vi "Main Target v3.vi"() -> ()   [LabVIEW 2018]
uses:
  Messages.ctl
  Target Logging Cluster.ctl
  Logging Data Cluster.ctl
  Target Logging Control Signals.ctl
  Target Logging Sensors.ctl
  Sensor Data.ctl
  <vilib>/Platform/TimedLoop/XDataNode/timing_clust.ctl
  <vilib>/Platform/TimedLoop/XDataNode/nitl_modes.ctl
  <vilib>/Platform/TimedLoop/XDataNode/wakeup.ctl
  Target IO Initialized Cluster.ctl
  <vilib>/myRIO/Instrument Drivers/Onboard IO/AI/typedefs/AI Reference.ctl
  <vilib>/myRIO/Common/Instrument Driver Framework/Utilities/typedefs/myRIO Generic Hardware Reference.ctl
  <vilib>/myRIO/Common/Instrument Driver Framework/Utilities/typedefs/Hardware Version Enum.ctl
  <vilib>/myRIO/Common/Instrument Driver Framework/Utilities/typedefs/myRIO v1.0 Reference.ctl
  <vilib>/myRIO/Common/Instrument Driver Framework/Utilities/typedefs/Generic FPGA Reference.ctl
  <vilib>/myRIO/Common/Instrument Driver Framework/myRIO v1.0/AI/typedefs/AI Channels List.ctl
  <vilib>/myRIO/Common/Instrument Driver Framework/myRIO v1.0/AI/typedefs/AI Channels Enum.ctl
  <vilib>/myRIO/Common/Instrument Driver Framework/Utilities/typedefs/Analog Scaling Constants List.ctl
  <vilib>/myRIO/Common/Instrument Driver Framework/Utilities/typedefs/Analog Scaling Constants.ctl
  <vilib>/myRIO/Instrument Drivers/Onboard IO/AO/typedefs/AO Reference.ctl
  <vilib>/myRIO/Common/Instrument Driver Framework/myRIO v1.0/AO/typedefs/AO Channels List.ctl
  <vilib>/myRIO/Common/Instrument Driver Framework/myRIO v1.0/AO/typedefs/AO Channels Enum.ctl
  <vilib>/myRIO/Instrument Drivers/Onboard IO/Encoder/typedefs/Encoder Reference.ctl
  <vilib>/myRIO/Common/Instrument Driver Framework/myRIO v1.0/Encoder/typedefs/Encoder Channels Enum.ctl
  <vilib>/myRIO/Instrument Drivers/Onboard IO/DIO/typedefs/DIO Reference.ctl
  <vilib>/myRIO/Common/Instrument Driver Framework/myRIO v1.0/DIO/typedefs/DIO Channels List.ctl
  <vilib>/myRIO/Common/Instrument Driver Framework/myRIO v1.0/DIO/typedefs/DIO Channels Enum.ctl
  <vilib>/myRIO/Common/Instrument Driver Framework/myRIO v1.0/DIO/vis/myRIO v1.0 Close DIO.vi
  <vilib>/myRIO/Common/Instrument Driver Framework/myRIO v1.0/Encoder/vis/myRIO v1.0 Close Encoder.vi
  <vilib>/myRIO/Common/Instrument Driver Framework/myRIO v1.0/AO/vis/myRIO v1.0 Close AO.vi
  <vilib>/myRIO/Common/Instrument Driver Framework/myRIO v1.0/AI/vis/myRIO v1.0 Close AI.vi
  <vilib>/myRIO/Common/Instrument Driver Framework/myRIO v1.0/UART/vis/myRIO v1.0 Close UART.vi
  <vilib>/myRIO/Common/Instrument Driver Framework/myRIO v1.0/DIO/vis/myRIO v1.0 Unreserve DIO.vi
  <vilib>/myRIO/Common/Instrument Driver Framework/myRIO v1.0/Encoder/vis/myRIO v1.0 Unreserve Encoder.vi
  <vilib>/myRIO/Common/Instrument Driver Framework/myRIO v1.0/AO/vis/myRIO v1.0 Unreserve AO.vi
  <vilib>/myRIO/Common/Instrument Driver Framework/myRIO v1.0/AI/vis/myRIO v1.0 Unreserve AI.vi
  <vilib>/myRIO/Common/Instrument Driver Framework/myRIO v1.0/DIO/vis/myRIO v1.0 Build MUX Configuration DIO.vi
  <vilib>/myRIO/Common/Instrument Driver Framework/myRIO v1.0/Resource Manager/vis/myRIO v1.0 Unreserve Channel List.vi
  <vilib>/myRIO/Common/Instrument Driver Framework/myRIO v1.0/Encoder/vis/myRIO v1.0 Build MUX Configuration Encoder.vi
  <vilib>/myRIO/Common/Instrument Driver Framework/myRIO v1.0/AO/vis/myRIO v1.0 Build MUX Configuration AO.vi
  <vilib>/myRIO/Common/Instrument Driver Framework/myRIO v1.0/AI/vis/myRIO v1.0 Build MUX Configuration AI.vi
  <vilib>/myRIO/Common/Instrument Driver Framework/myRIO v1.0/Resource Manager/vis/myRIO v1.0 Create Configuration List.vi
  <vilib>/myRIO/Common/Instrument Driver Framework/myRIO v1.0/Resource Manager/vis/myRIO v1.0 Unreserve Channel.vi
  <vilib>/myRIO/Common/Instrument Driver Framework/myRIO v1.0/Resource Manager/vis/myRIO v1.0 Build Mutex Name.vi
  <vilib>/Utility/error.llb/Error Cluster From Error Code.vi
  <vilib>/myRIO/Common/Instrument Driver Framework/myRIO v1.0/DIO/vis/myRIO v1.0 Write DIO.vi
  <vilib>/myRIO/Common/Instrument Driver Framework/myRIO v1.0/DIO/vis/myRIO v1.0 Shutdown DIO.vi
  <vilib>/myRIO/Common/Instrument Driver Framework/myRIO v1.0/Resource Manager/vis/myRIO v1.0 Configure IO.vi
  <vilib>/myRIO/Common/Instrument Driver Framework/Utilities/vis/Configuration Manager.vi
  <vilib>/myRIO/Common/Instrument Driver Framework/Utilities/vis/IO Manager.vi
  <vilib>/myRIO/Common/Instrument Driver Framework/myRIO v1.0/myRIO v1.0 Close.vi
  <vilib>/myRIO/Common/Instrument Driver Framework/myRIO v1.0/Encoder/vis/myRIO v1.0 Shutdown Encoder.vi
  <vilib>/myRIO/Common/Instrument Driver Framework/myRIO v1.0/IRQ/vis/myRIO v1.0 Reserve IRQ.vi
  <vilib>/myRIO/Common/Instrument Driver Framework/Utilities/vis/FPGA Ref Manager.vi
  <vilib>/myRIO/Common/Instrument Driver Framework/myRIO v1.0/AO/vis/myRIO v1.0 Write AO.vi
  <vilib>/myRIO/Common/Instrument Driver Framework/myRIO v1.0/myRIO v1.0 Reset FPGA.vi
  <vilib>/myRIO/Common/Instrument Driver Framework/myRIO v1.0/IRQ/vis/myRIO v1.0 IRQ Info FGV.vi
  <vilib>/myRIO/Common/Instrument Driver Framework/myRIO v1.0/IRQ/vis/myRIO v1.0 Timer IRQ Info FGV.vi
  <vilib>/myRIO/Common/Instrument Driver Framework/myRIO v1.0/IRQ/vis/myRIO v1.0 ISR Agent.vi
  <vilib>/platform/TimedLoop/XDataNode/XDataNode.xnode
  <vilib>/Platform/TimedLoop/XDataNode/XDNodeRunTimeDep.lvlib
  <vilib>/myRIO/Instrument Drivers/Onboard IO/AI/AI.lvlib
  <vilib>/myRIO/Instrument Drivers/Onboard IO/AO/AO.lvlib
  <vilib>/myRIO/Instrument Drivers/Onboard IO/Encoder/Encoder.lvlib
  <vilib>/myRIO/Instrument Drivers/IRQ/IO IRQ/IO IRQ.lvlib
  <vilib>/myRIO/Instrument Drivers/Onboard IO/DIO/DIO.lvlib
  <vilib>/myRIO/Instrument Drivers/Utilities/Utilities.lvlib
panel:
  out "Number of Late Loops":dbl
  out "UART Error Out":errorcluster
  out "Data Logging Error":errorcluster
  out "Period":u32
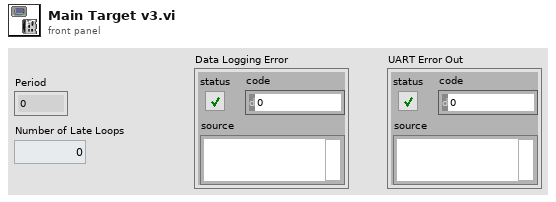
[diagram p1: front panel]
types:
  T1 = typedef "Target Logging Cluster.ctl" = cluster{"Valid for Logging?":bool, "Data":T2}
  T2 = typedef "Logging Data Cluster.ctl" = cluster{"Control Signals":T3, "Target Sensors":T4}
  T3 = typedef "Target Logging Control Signals.ctl" = cluster{"Phi":dbl, "Gait %":dbl, "ILC Desired Ankle Angle":dbl, "Desired Motor Current":dbl, "Transmission Ratio":dbl, "Passive Torque Estimate":dbl, "Torque Reference":dbl, "Left HS?":bool, "Left HS State":u32, "Right HS?":bool, "Right HS State":u32, "dGRF L":dbl, "dGRF R":dbl, "GRF L (filt) ":dbl, "GRF R (filt)":dbl}
  T4 = typedef "Target Logging Sensors.ctl" = cluster{"Sensors":T5}
  T5 = typedef "Sensor Data.ctl" = cluster{"Motor Current":dbl, "Motor Velocity":dbl, "Ankle Encoder Angle":dbl, "GRF L":dbl, "GRF R":dbl, "Index pulse?":bool, "Roll":dbl, "Pitch":dbl, "Yaw":dbl, "Thigh Angle":dbl}
  T6 = typedef "Messages.ctl" = enum16{"Stop", "Activate/Deactivate Controller", "Log Data", "FF Control Gain Change", "F Thr Change", "dF Thr Change", "Bias Current Change", "Filename Change", "Logging Duration Change", "Phi 1 Change", "Phi End Change", "Phi Remainder Change", "Cutoff Freq Changed", "Control Gain Changed", "Num Phi Param Samples Changed"}
  T7 = typedef "XDNodeRunTimeDep.lvlib/timing_clust.ctl" = cluster{"Expected End [f-1]":u64, "Actual End [f-1]":u64, "Finished Late? [f-1]":bool, "Expected End [i-1]":u64, "Actual End [i-1]":u64, "Finished Late? [i-1]":bool, "Expected Start [i]":u64, "Actual Start [i]":u64, "Expected Start [f]":u64, "Actual Start [f]":u64, "Source Name":string, "Structure Name":string, "Period":i64, "Deadline":i64, "Offset":i64, "Start":i64, "Priority":i32, "Timeout":i32, "Mode":T8, "Wakeup Reason":T9, "Error":errorcluster, "Source Type":string, "Secondary Source Type":string, "Global End Time":u64, "Global Start Time":u64, "Frame Duration":u64, "Iteration Duration":u64, "Assigned CPU":i32, "I/O Scan Engine Mode":u32}
  T8 = typedef "XDNodeRunTimeDep.lvlib/nitl_modes.ctl" = enum32{"No Change", "Process missed periods, maintain original phase", "Discard missed periods, maintain original phase", "Process missed periods, ignore original phase", "Discard missed periods, ignore original phase"}
  T9 = typedef "XDNodeRunTimeDep.lvlib/wakeup.ctl" = enum32{"Normal", "Aborted", "Asynchronous wakeup", "Timing source error", "Timed loop error", "Timeout"}
  T10 = typedef "Target IO Initialized Cluster.ctl" = cluster{"AI Ref Out":T11, "AO Ref Out":T20, "Encoder Ref Out":T23, "UART resource name out":refnum<visa-resource-name>, "DIO Ref Out":T25}
  T11 = typedef "AI.lvlib/AI Reference.ctl" = cluster{"myRIO Reference":T12, "AI Channels List":T16, "AI Scaling Constants List":T18}
  T12 = typedef "myRIO Generic Hardware Reference.ctl" = cluster{"myRIO Model":T13, "myRIO Hardware Reference":T14}
  T13 = typedef "Hardware Version Enum.ctl" = enum16{"Unknown", "myRIO-1900", "myRIO-1950", "roboRIO", "NI ELVIS RIO CM", "ELVIS III"}
  T14 = typedef "myRIO v1.0 Reference.ctl" = cluster{"Generic FPGA Reference":T15, "Allow multiple opens":bool}
  T15 = typedef "Generic FPGA Reference.ctl" = refnum<k20>
  T16 = typedef "AI Channels List.ctl" = T17[]
  T17 = typedef "AI Channels Enum.ctl" = enum16{"Not Connected", "AudioIn/Left", "AudioIn/Right", "C/AI0", "C/AI1", "A/AI0", "A/AI1", "A/AI2", "A/AI3", "A/AI4", "A/AI5", "A/AI6", "A/AI7", "B/AI0", "B/AI1", "B/AI2", "B/AI3", "B/AI4", "B/AI5", "B/AI6", "B/AI7", "AI/AI0", "AI/AI1", "AI/AI2", "AI/AI3", "A/AI0 (DIFF)", "A/AI1 (DIFF)", "A/AI2 (DIFF)", "A/AI3 (DIFF)", "B/AI0 (DIFF)", "B/AI1 (DIFF)", "B/AI2 (DIFF)", "B/AI3 (DIFF)"}
  T18 = typedef "Analog Scaling Constants List.ctl" = T19[]
  T19 = typedef "Analog Scaling Constants.ctl" = cluster{"LSB Weight (Volts)":dbl, "Offset (Volts)":dbl, "Signed?":bool}
  T20 = typedef "AO.lvlib/AO Reference.ctl" = cluster{"myRIO Reference":T12, "AO Channel List":T21, "AO Scaling Constant List":T18}
  T21 = typedef "AO Channels List.ctl" = T22[]
  T22 = typedef "AO Channels Enum.ctl" = enum16{"Not Connected", "AudioOut/Left", "AudioOut/Right", "C/AO0", "C/AO1", "A/AO0", "A/AO1", "B/AO0", "B/AO1"}
  T23 = typedef "Encoder.lvlib/Encoder Reference.ctl" = cluster{"myRIO Reference":T12, "Encoder Channels Enum":T24}
  T24 = typedef "Encoder Channels Enum.ctl" = enum16{"Not Connected", "C/ENC0", "C/ENC1", "A/ENC", "A/ENC0", "A/ENC1", "A/ENC2", "A/ENC3", "A/ENC4", "A/ENC5", "A/ENC6", "A/ENC7", "A/ENC8", "A/ENC9", "B/ENC", "B/ENC0", "B/ENC1", "B/ENC2", "B/ENC3", "B/ENC4", "B/ENC5", "B/ENC6", "B/ENC7", "B/ENC8", "B/ENC9", "DIO/ENC0", "DIO/ENC1", "DIO/ENC2", "DIO/ENC3", "DIO/ENC4"}
  T25 = typedef "DIO.lvlib/DIO Reference.ctl" = cluster{"myRIO Reference":T12, "DIO Channels List":T26}
  T26 = typedef "DIO Channels List.ctl" = T27[]
  T27 = typedef "DIO Channels Enum.ctl" = enum16{"Not Connected", "C/DIO0", "C/DIO1", "C/DIO2", "C/DIO3", "C/DIO4", "C/DIO5", "C/DIO6", "C/DIO7", "A/DIO0", "A/DIO1", "A/DIO2", "A/DIO3", "A/DIO4", "A/DIO5", "A/DIO6", "A/DIO7", "A/DIO8", "A/DIO9", "A/DIO10", "A/DIO11", "A/DIO12", "A/DIO13", "A/DIO14", "A/DIO15", "A/DIO16", "A/DIO17", "A/DIO18", "A/DIO19", "B/DIO0", "B/DIO1", "B/DIO2", "B/DIO3", "B/DIO4", "B/DIO5", "B/DIO6", "B/DIO7", "B/DIO8", "B/DIO9", "B/DIO10", "B/DIO11", "B/DIO12", "B/DIO13", "B/DIO14", "B/DIO15", "B/DIO16", "B/DIO17", "B/DIO18", "B/DIO19", "LED0", "LED1", "LED2", "LED3", "Button0", "DIO/DIO0", "DIO/DIO1", "DIO/DIO2", "DIO/DIO3", "DIO/DIO4", "DIO/DIO5", "DIO/DIO6", "DIO/DIO7", "DIO/DIO8", "DIO/DIO9", "SPI/CS0", "SPI/CS1", "SPI/CS2", "SPI/CS3", "LED RADIO (Green)", "LED RADIO (Red)", "LED COMM (Green)", "LED COMM (Red)", "LED MODE (Green)", "LED MODE (Red)"}
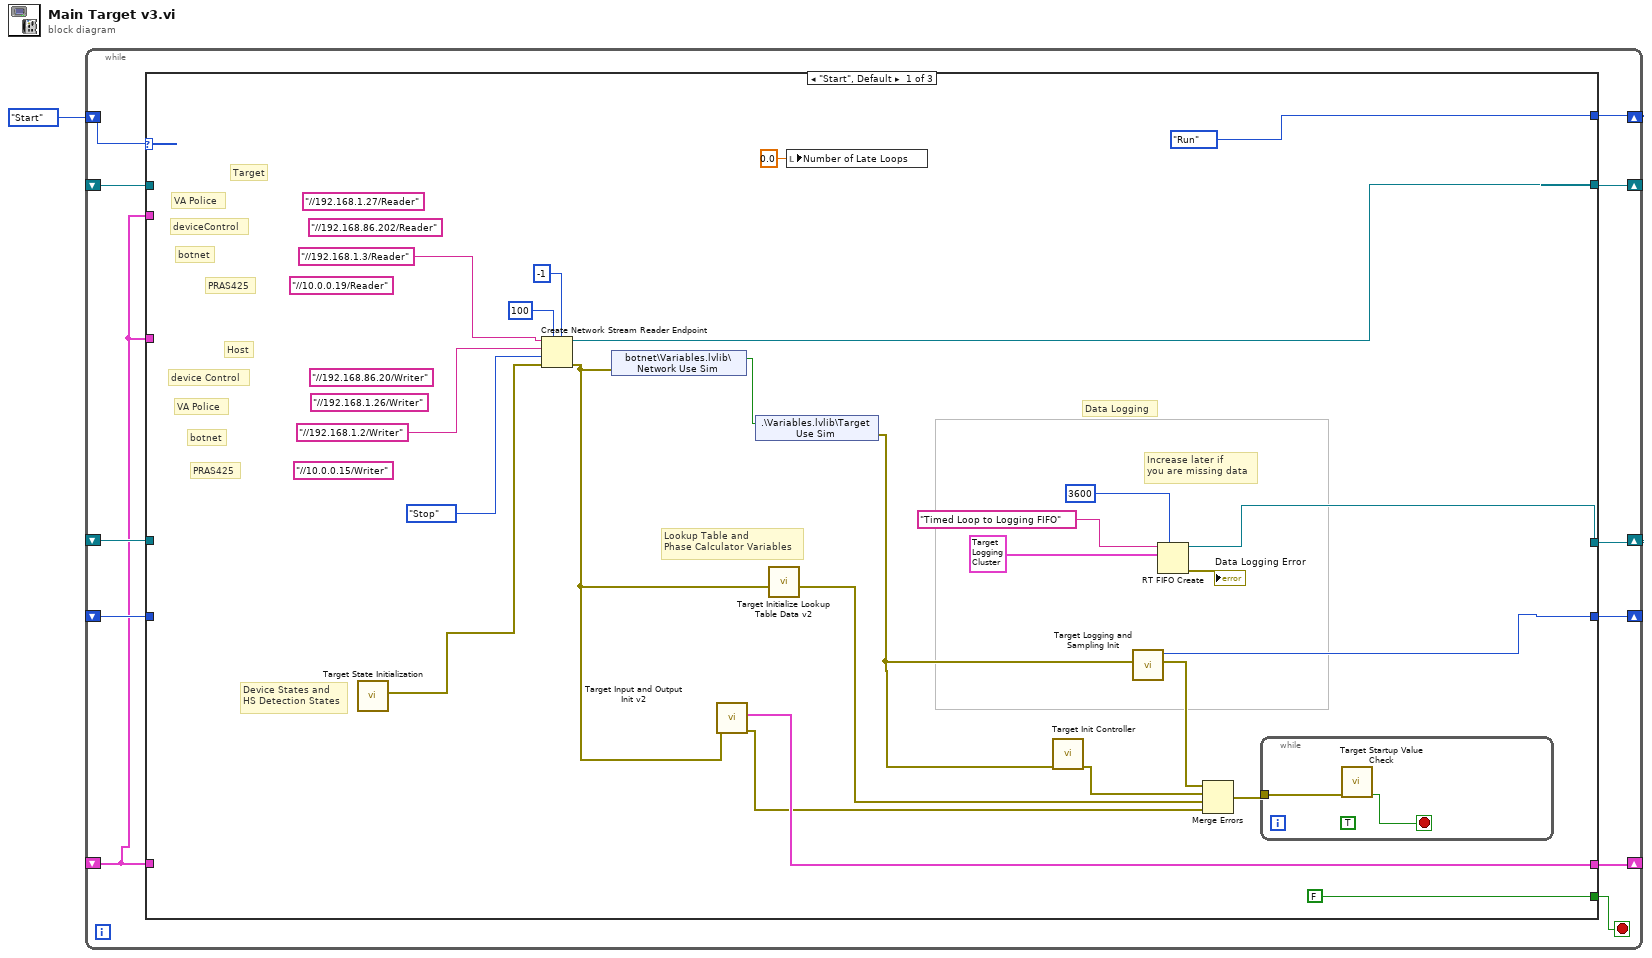
[diagram p0: block diagram]
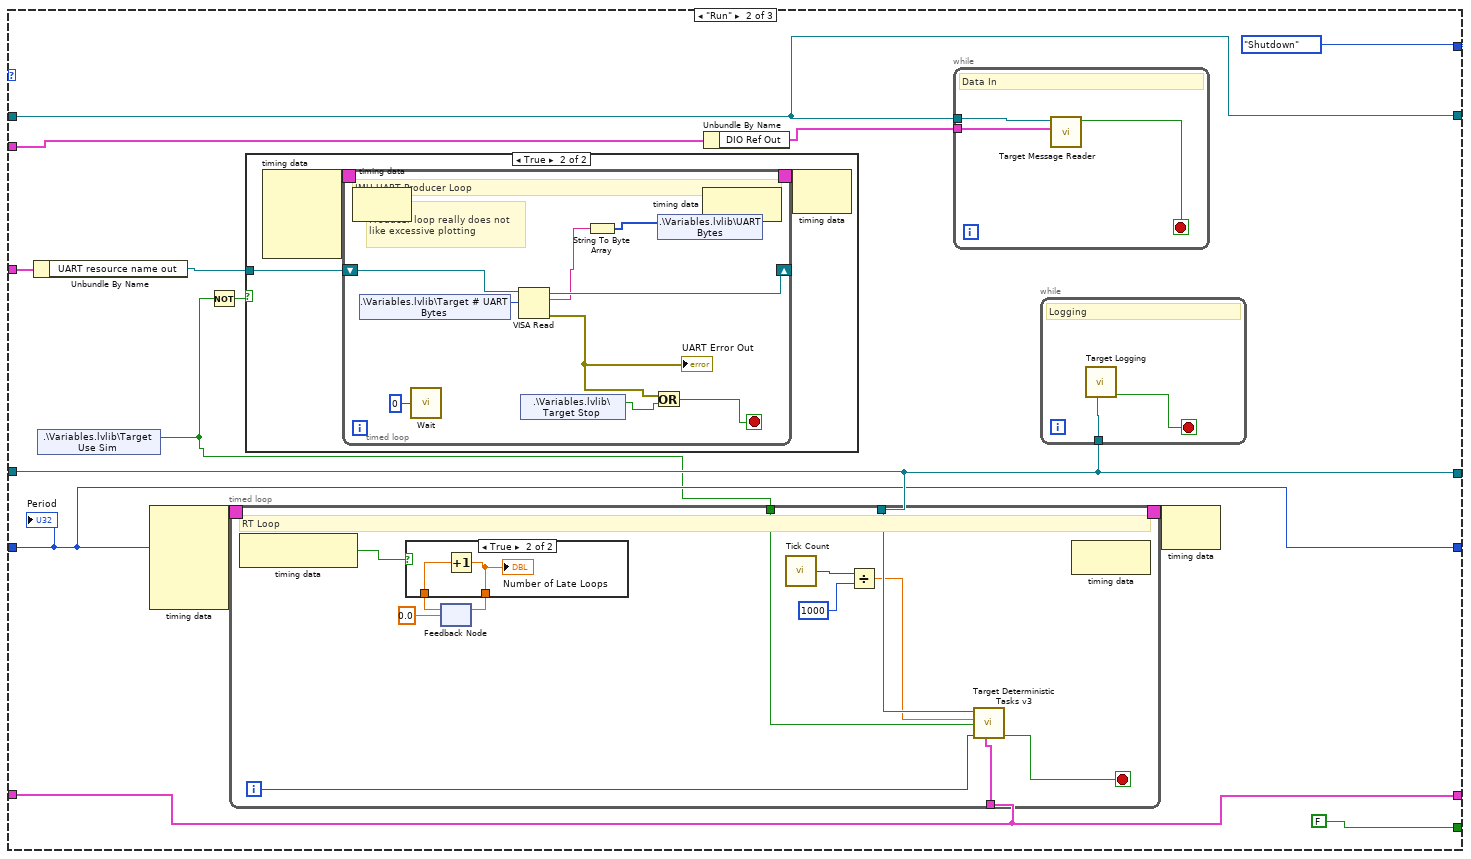
[diagram p2: hidden frame]
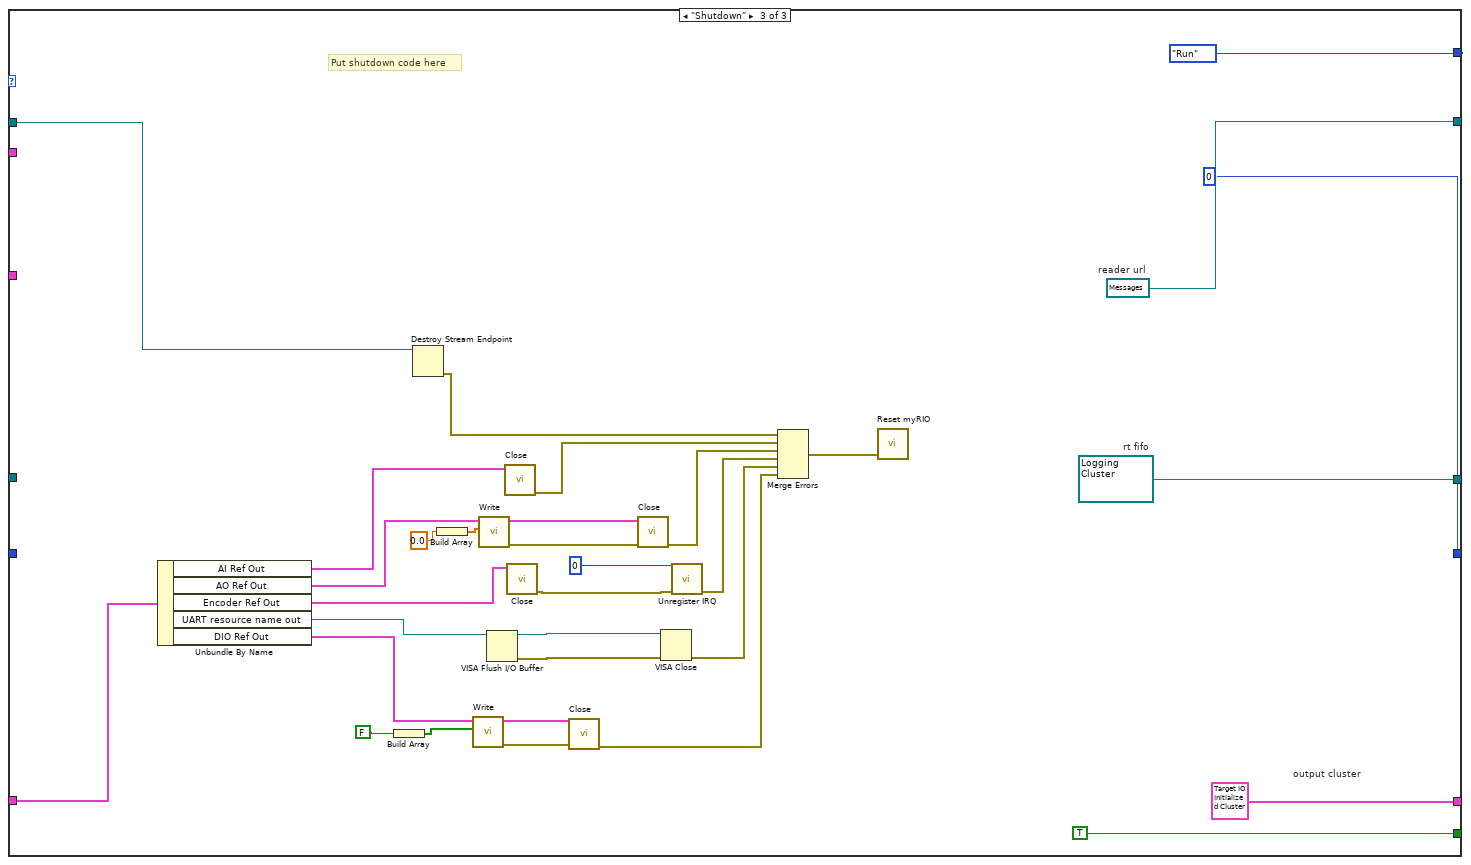
[diagram p5: hidden frame]
diagram:
  n1 = while {
    shift-right: [w11] -> _
    shift-left: enum16{"Start", "Run", "Shutdown"}."Start" -> [w12]
    shift-right: [w9] -> _
    shift-left: _ -> [w8]
    shift-right: [w6] -> _
    shift-left: _ -> [w5]
    shift-right: [w4] -> _
    shift-left: _ -> [w7]
    shift-right: [w3] -> _
    shift-left: _ -> [w2]
    stop <- w10 stop-if-true
    n2 = case shown="\"Start\", Default" w12 {
      tunnel: [FALSE FALSE TRUE] -> w10
      tunnel: [enum16{"Start", "Run", "Shutdown"}."Run" enum16{"Start", "Run", "Shutdown"}."Shutdown" enum16{"Start", "Run", "Shutdown"}."Run"] -> w11
      tunnel: [w33 w49 w125] -> w9
      tunnel: w8 -> [_ w49 w126]
      tunnel: w7 -> [_ w47 _]
      tunnel: [w32 w48 w124] -> w6
      tunnel: w5 -> [_ w48 _]
      tunnel: [w27 w47 u32 0 ("UInt32")] -> w4
      tunnel: [w26 w46 w122] -> w3
      tunnel: w2 -> [_ w46 w121]
      tunnel: w2 -> [_ w45 _]
      tunnel: w2 -> [_ w43 _]
      frame "Start", Default {
        (unwired) "//10.0.0.19/Reader" ("writer name")
        (unwired) "//10.0.0.15/Writer" ("writer name")
        (unwired) "//192.168.1.26/Writer" ("writer name")
        (unwired) "//192.168.1.27/Reader" ("reader url")
        (unwired) "//192.168.86.20/Writer" ("writer name")
        (unwired) "//192.168.86.202/Reader" ("reader url")
        # "PRAS425"
        # "PRAS425"
        # "botnet"
        # "botnet"
        # "Device States and\nHS Detection States"
        # "Data Logging"
        # "Increase later if \nyou are missing data"
        # "device Control"
        # "VA Police"
        # "deviceControl"
        # "VA Police"
        # "Host"
        # "Target"
        # "Lookup Table and \nPhase Calculator Variables"
        n3 = call "Target State Initialization.vi"() -> ("error out"=w24:errorcluster)  [unwired: 11 in]
        n4 = Create Network Stream Reader Endpoint(5:-1 ("timeout in ms (-1)"), 7:100 ("reader buffer size"), 8:w24, 9:Messages."Stop" ("Messages"), 10:"//192.168.1.2/Writer" ("writer name"), 11:"//192.168.1.3/Reader" ("reader url")) -> (0:w17:errorcluster, 3:w33:refnum<k21>)  [unwired: 1 in]
        n5 = shared-variable "botnet\\Variables.lvlib\\Network Use Sim"(error in=w17) -> (w19:bool)  [unwired: 1 out]
        n6 = call "Target Input and Output Init v2.vi"("error in (no error)"=w17) -> ("error out"=w16:errorcluster, "output cluster"=w26:T10)  [unwired: 9 in]
        n7 = shared-variable ".\\Variables.lvlib\\Target Use Sim"(w19) -> (error out=w18:errorcluster)  [unwired: 1 in]
        n8 = call "Target Initialize Lookup Table Data v2.vi"("error in (no error)"=w17) -> ("error out"=w15:errorcluster)  [unwired: 10 in]
        n9 = local write "Number of Late Loops"(0.0 ("Number of Late Loops")) -> ()
        n10 = call "Target Init Controller.vi"("error in (no error)"=w18) -> ("error out"=w21:errorcluster)  [unwired: 10 in]
        n11 = call "Target Logging and Sampling Init.vi"("error in (no error)"=w18) -> ("error out"=w22:errorcluster, "Sampling Period (microsec)"=w27:i32)  [unwired: 9 in]
        n12 = RT FIFO Create(0:"Timed Loop to Logging FIFO" ("name (unnamed)"), 1:T1 {"Valid for Logging?"=FALSE, "Data"={"Control Signals"={"Phi"=0.0, "Gait %"=0.0, "ILC Desired Ankle Angle"=0.0, "Desired Motor Current"=0.0, "Transmission Ratio"=0.0, "Passive Torque Estimate"=0.0, "Torque Reference"=0.0, "Left HS?"=FALSE, "Left HS State"=0, "Right HS?"=FALSE, "Right HS State"=0, "dGRF L"=0.0, "dGRF R"=0.0, "GRF L (filt) "=0.0, "GRF R (filt)"=0.0}, "Target Sensors"={"Sensors"={"Motor Current"=0.0, "Motor Velocity"=0.0, "Ankle Encoder Angle"=0.0, "GRF L"=0.0, "GRF R"=0.0, "Index pulse?"=FALSE, "Roll"=0.0, "Pitch"=0.0, "Yaw"=0.0, "Thigh Angle"=0.0}}}} ("Logging Cluster"), 4:u32 3600 ("size (10)")) -> (8:w32:refnum<k33>, 11:→"Data Logging Error":errorcluster)  [unwired: 5 in, 1 out]
        n13 = Merge Errors(w22, w21, w15, w16) -> (w23:errorcluster)
        n14 = while {
          tunnel: w23 -> [w39]
          stop <- w38 stop-if-true
          (unwired) TRUE
          n15 = call "Target Startup Value Check.vi"("error in (no error)"=w39) -> ("Ok to run?"=w38:bool)  [unwired: 10 in]
        }
      }
      frame "Run" {
        n16 = Unbundle By Name(w45) -> ("UART resource name out"=w44:refnum<visa-resource-name>)
        n17 = shared-variable ".\\Variables.lvlib\\Target Use Sim"() -> (w40:bool)  [unwired: 1 in, 1 out]
        n18 = node-c288(w47) -> (w51:T7)  [unwired: 4 in]
        n19 = Not(x=w40) -> (.not. x?=w41:bool)
        n20 = timed-loop {
          timing: w51 -> [_]
          timing-out: [_] -> w50
          tunnel: w48 -> [w81]
          tunnel: w46 -> [w77]
          tunnel: w40 -> [w72]
          i -> [w82]
          stop <- w83 stop-if-true
          # "RT Loop"
          n21 = node-c288() -> (w76:bool)  [unwired: 1 in]
          n22 = feedback #1(0.0) -> (w74:dbl)
          n23 = case shown="True" w76 {
            tunnel: [w84 w85] -> w75
            tunnel: w74 -> [w84 w86]
            frame False {
            }
            frame True {
              n24 = Increment(x=w86) -> (x+1=w85:dbl)
              "Number of Late Loops" <- w85
            }
          }
          n25 = feedback-in #1(w75) -> ()
          n26 = call "Tick Count"() -> ("Tick Count(mSec)"=w80:u32)
          n27 = Divide(x=w80, y=u32 1000) -> (x/y=w78:dbl)
          n28 = call "Target Deterministic Tasks v3.vi"("I/O Cluster"=w77, "Loop Iteration"=w82, "Use simulation data?"=w72, "Current Time (s)"=w78, "rt fifo"=w81) -> ("Timed Loop Stop"=w83:bool)  [unwired: 6 in]
          n29 = node-c288() -> ()  [unwired: 1 in, 1 out]
        }
        n30 = case shown="True" w41 {
          tunnel: w44 -> [_ w56]
          frame False {
          }
          frame True {
            n31 = node-c288() -> (w55:T7)  [unwired: 4 in]
            n32 = timed-loop {
              shift-right: [w65] -> _
              shift-left: w56 -> [w64]
              timing: w55 -> [_]
              timing-out: [_] -> w54
              stop <- w57 stop-if-true
              # "NOTE:\nProducer loop really does not\nlike excessive plotting"
              # "IMU UART Producer Loop"
              n33 = node-c288() -> ()  [unwired: 1 in, 1 out]
              n34 = shared-variable ".\\Variables.lvlib\\Target # UART Bytes"() -> (w58:u8)  [unwired: 1 in, 1 out]
              n35 = call "Wait"("Count(uSec)"=u32 0) -> ()  [unwired: 1 out]
              n36 = VISA Read(VISA resource name=w64, byte count=w58) -> (VISA resource name out=w65:refnum<visa-resource-name>, read buffer=w63:string, error out=w61:errorcluster)  [unwired: 1 in, 1 out]
              "UART Error Out" <- w61
              n37 = shared-variable ".\\Variables.lvlib\\Target Stop"() -> (w59:bool)  [unwired: 1 in, 1 out]
              n38 = String To Byte Array(string=w63) -> (unsigned byte array=w62:u8[])
              n39 = Or(x=w61, y=w59) -> (x .or. y?=w57:bool)
              n40 = shared-variable ".\\Variables.lvlib\\UART Bytes"(w62) -> ()  [unwired: 1 in, 1 out]
              n41 = node-c288() -> ()  [unwired: 1 in, 1 out]
            }
            n42 = node-c288(w54) -> ()  [unwired: 1 out]
          }
        }
        n43 = Unbundle By Name(w43) -> ("DIO Ref Out"=w42:T25)
        n44 = while {
          tunnel: w49 -> [w96]
          tunnel: w42 -> [w94]
          stop <- w95 stop-if-true
          # "Data In"
          n45 = call "Target Message Reader.vi"("DIO Ref In"=w94, "reader url"=w96) -> ("Stop"=w95:bool)  [unwired: 9 in]
        }
        n46 = while {
          tunnel: w48 -> [w70]
          stop <- w71 stop-if-true
          # "Logging"
          n47 = call "Target Logging.vi"("rt fifo"=w70) -> ("Stop Loop"=w71:bool)  [unwired: 10 in]
        }
        n48 = node-c288(w50) -> ()  [unwired: 1 out]
        "Period" <- w47
      }
      frame "Shutdown" {
        w122 = T10 {"AI Ref Out"={"myRIO Reference"={"myRIO Model"=enum."Unknown", "myRIO Hardware Reference"={"Generic FPGA Reference"=refnum, "Allow multiple opens"=FALSE}}, "AI Channels List"=[], "AI Scaling Constants List"=[]}, "AO Ref Out"={"myRIO Reference"={"myRIO Model"=enum."Unknown", "myRIO Hardware Reference"={"Generic FPGA Reference"=refnum, "Allow multiple opens"=FALSE}}, "AO Channel List"=[], "AO Scaling Constant List"=[]}, "Encoder Ref Out"={"myRIO Reference"={"myRIO Model"=enum."Unknown", "myRIO Hardware Reference"={"Generic FPGA Reference"=refnum, "Allow multiple opens"=FALSE}}, "Encoder Channels Enum"=enum."Not Connected"}, "UART resource name out"="", "DIO Ref Out"={"myRIO Reference"={"myRIO Model"=enum."Unknown", "myRIO Hardware Reference"={"Generic FPGA Reference"=refnum, "Allow multiple opens"=FALSE}}, "DIO Channels List"=[]}}  # output cluster
        w124 = refnum<k33> refnum  # rt fifo
        w125 = refnum<k21> refnum items=["Stop", "Activate/Deactivate Controller", "Log Data", "FF Control Gain Change", "F Thr Change", "dF Thr Change", "Bias Current Change", "Filename Change", "Logging Duration Change", "Phi 1 Change", "Phi End Change", "Phi Remainder Change", "Cutoff Freq Changed", "Control Gain Changed", "Num Phi Param Samples Changed"]  # reader url
        # "Put shutdown code here"
        n49 = Unbundle By Name(w121) -> ("AI Ref Out"=w120:T11, "AO Ref Out"=w101:T20, "Encoder Ref Out"=w117:T23, "UART resource name out"=w114:refnum<visa-resource-name>, "DIO Ref Out"=w113:T25)
        n50 = Build Array(FALSE) -> (w112:bool[])
        n51 = Destroy Stream Endpoint(11:w126) -> (0:w107:errorcluster)  [unwired: 1 in]
        n52 = Build Array(0.0 ("element")) -> (w97:dbl[])
        n53 = call <vilib>:"Write.vi"("Values"=w112, "DIO Ref In"=w113) -> ("error out"=w109:errorcluster, "DIO Ref Out"=w110:T25)  [unwired: 7 in]
        n54 = call <vilib>:"Write.vi"("Values"=w97, "AO Ref In"=w101) -> ("error out"=w99:errorcluster, "AO Ref Out"=w100:T20)  [unwired: 7 in]
        n55 = VISA Flush I/O Buffer(VISA resource name=w114) -> (VISA resource name out=w116:refnum<visa-resource-name>, error out=w115:errorcluster)  [unwired: 2 in]
        n56 = call <vilib>:"Close.vi"("AI Ref In"=w120) -> ("error out"=w106:errorcluster)  [unwired: 10 in]
        n57 = call <vilib>:"Close.vi"("Encoder Ref In"=w117) -> ("error out"=w118:errorcluster)  [unwired: 10 in]
        n58 = call <vilib>:"Close.vi"("error in (no error)"=w109, "DIO Ref In"=w110) -> ("error out"=w102:errorcluster)  [unwired: 9 in]
        n59 = call <vilib>:"Close.vi"("error in (no error)"=w99, "AO Ref In"=w100) -> ("error out"=w105:errorcluster)  [unwired: 9 in]
        n60 = VISA Close(VISA resource name=w116, error in (no error)=w115) -> (error out=w103:errorcluster)
        n61 = call <vilib>:"Unregister IRQ.vi"("error in (no error)"=w118, "IRQ Number"=0) -> ("error out"=w104:errorcluster)  [unwired: 9 in]
        n62 = Merge Errors(w107, w106, w105, w104, w103, w102) -> (w108:errorcluster)
        n63 = call <vilib>:"Reset myRIO.vi"("error in (no error)"=w108) -> ()  [unwired: 10 in, 1 out]
      }
    }
  }
